vi "Split Statement.vi"(6 "error in (no error)":errorcluster, 10 "Statement":string) -> (3 "Tokens":string[](array[string]), 4 "error out":errorcluster)   [LabVIEW 2017]
uses:
  <vilib>/Utility/error.llb/Error Cluster From Error Code.vi
  <vilib>/ErrorRing/Error Ring.xnode
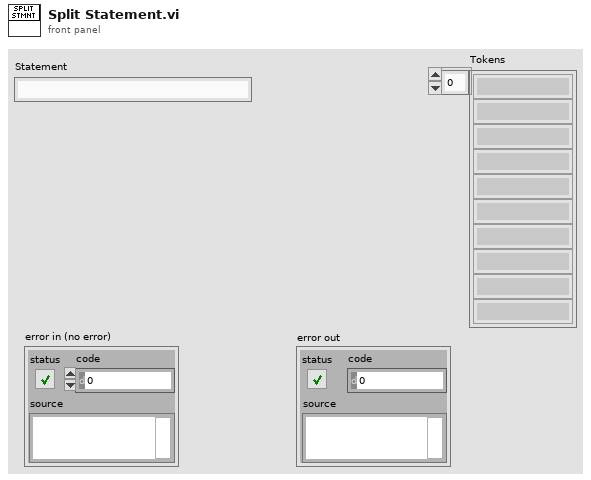
[diagram p1: front panel]
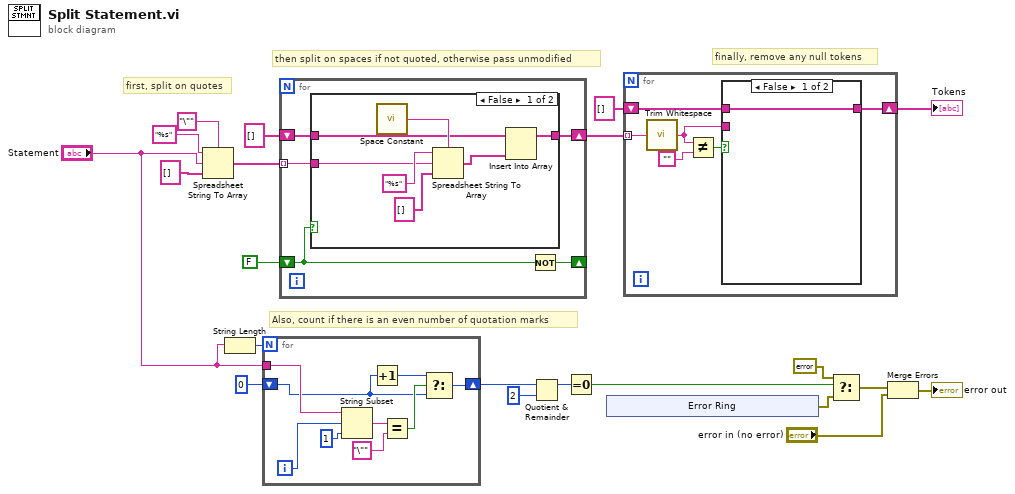
[diagram p0: block diagram]
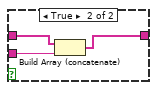
[diagram p2: hidden frame]
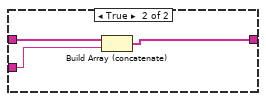
[diagram p3: hidden frame]
diagram:
  # "finally, remove any null tokens"
  # "then split on spaces if not quoted, otherwise pass unmodified"
  # "first, split on quotes"
  # "Also, count if there is an even number of quotation marks"
  n1 = Spreadsheet String To Array(delimiter (Tab)="\"", format string="%s", spreadsheet string="Statement", array type (2D Dbl)=string[] []) -> (array=w18:string[])
  n2 = String Length(string="Statement") -> (length=w11:i32)
  n3 = for {
    N: w11 -> [_]
    tunnel: "Statement" -> [w30]
    shift-right: [w24] -> w9
    shift-left: 0 -> [w22]
    i -> [w28]
    n4 = String Subset(string=w30, offset (0)=w28, length (rest)=1 ("length (rest)")) -> (substring=w26:string)
    n5 = Increment(x=w22) -> (x+1=w23:i32)
    n6 = Equal?(x=w26, y="\"") -> (x = y?=w25:bool)
    n7 = Select(t=w23, s=w25, f=w22) -> (s? t:f=w24:i32)
  }
  n8 = for {
    tunnel: w18 -> [w33] mode=indexing
    shift-right: [w35] -> _
    shift-left: FALSE -> [w34]
    shift-right: [w31] -> w14
    shift-left: string[] [] -> [w32]
    n9 = case shown="False" w34 {
      tunnel: w33 -> [w40 w44]
      tunnel: w32 -> [w38 w45]
      tunnel: [w37 w43] -> w31
      frame False {
        n10 = call <vilib>:"Space Constant.vi"() -> ("String"=w39:string)
        n11 = Spreadsheet String To Array(delimiter (Tab)=w39, format string="%s", spreadsheet string=w40, array type (2D Dbl)=string[] []) -> (array=w36:string[])
        n12 = Insert Into Array(array=w38, new element=w36) -> (w37:string[])  [unwired: 1 in]
      }
      frame True {
        n13 = Build Array (concatenate)(w45, w44) -> (w43:string[])
      }
    }
    n14 = Not(x=w34) -> (.not. x?=w35:bool)
  }
  n15 = Quotient & Remainder(x=w9, y=2) -> (x-y*floor(x/y)=w7:i32)  [unwired: 1 out]
  n16 = Equal To 0?(x=w7) -> (x = 0?=w6:bool)
  n17 = xnode "Error Ring"() -> ("error out"=w5:errorcluster)
  n18 = for {
    shift-right: [w46] -> w13
    shift-left: string[] [] -> [w49]
    tunnel: w14 -> [w51] mode=indexing
    n19 = call <vilib>:"Trim Whitespace.vi"("string"=w51) -> ("trimmed string"=w47:string)  [unwired: 1 in]
    n20 = Not Equal?(x=w47, y="") -> (x != y?=w48:bool)
    n21 = case shown="False" w48 {
      tunnel: w49 -> [w52 w55]
      tunnel: w47 -> [_ w54]
      tunnel: [w52 w53] -> w46
      frame False {
      }
      frame True {
        n22 = Build Array (concatenate)(w55, w54) -> (w53:string[])
      }
    }
  }
  "Tokens" <- w13
  n23 = Select(t=errorcluster {"status"=FALSE, "code"=0, "source"=""}, s=w6, f=w5) -> (s? t:f=w2:errorcluster)
  n24 = Merge Errors(w2, "error in (no error)") -> (→"error out":errorcluster)
